vi "Send_string.vi"(8 "error in":errorcluster, 9 "flags_":i32, 10 "data":string, 11 "socket in":refnum<class "Socket.lvclass">) -> (0 "error out":errorcluster, 3 "socket out":refnum<class "Socket.lvclass">)   [LabVIEW 2025, in "ZeroMQ.lvlib" / "Socket.lvclass"]
doc: "Add the binary string <b>data</b> (the NULL value \\0 is permitted) to the output queue of the socket <b>socket in</b>.\n\nIf this message is part of a larger multi-component message and there are more parts to follow, then set <b>more?</b> to True.\n\nNote that when this call returns the message will likely <b>not have been sent yet</b> as it has only been placed in the queue for sending.\n\nDetailed API documentation: http://api.zeromq.org/3-2:zmq-send"
uses:
  Socket.lvclass
  Socket.lvclass/Socket.ctl
  libzmq-v143-mt-4_3_6/LibZMQ.lvlib
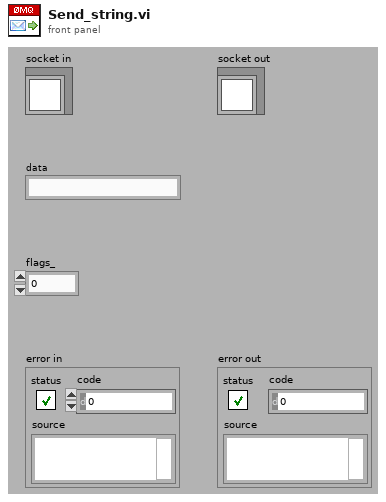
[diagram p1: front panel]
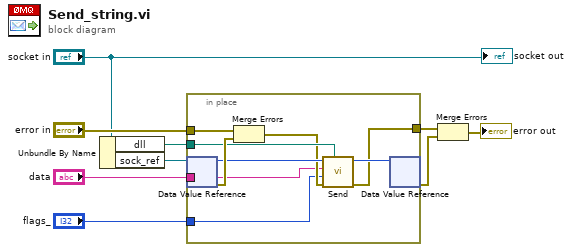
[diagram p0: block diagram]
diagram:
  n1 = Unbundle By Name("socket in") -> ("dll"=w2:path, "sock_ref"=w5:refnum<data-value>)
  n2 = in-place {
    in-place-border: "error in" -> [w18]
    in-place-border: "data" -> [w11]
    in-place-border: [w12] -> w7
    in-place-border: w2 -> [w16]
    in-place-border: "flags_" -> [w10]
    n3 = in-place-dvr #1(w5) -> (w15:u64, w17:errorcluster)
    n4 = Merge Errors(w18, w17) -> (w13:errorcluster)
    n5 = call "Send.vi"("path override"=w16, "error in (no error)"=w13, "flags_"=w10, "buf"=w11, "s"=w15) -> ("error out"=w12:errorcluster, "s_"=w14:u64)  [unwired: 5 in]
    n6 = in-place-dvr #1(w14) -> (w3:errorcluster)  [unwired: 1 out]
  }
  n7 = Merge Errors(w7, w3) -> (→"error out":errorcluster)
  "socket out" <- "socket in"
